vi "Correct_Position_info_7HP.vi"() -> (0 "error out":errorcluster, 4 "Path":path)   [LabVIEW 2018]
panel:
  out "File Changed":bool
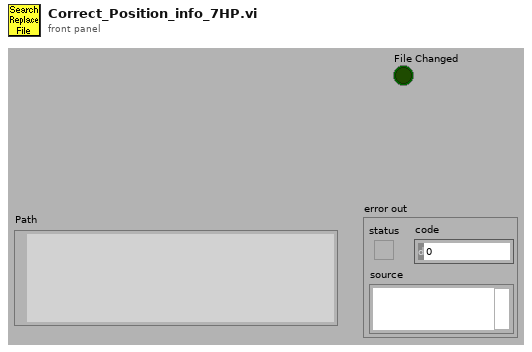
[diagram p1: front panel]
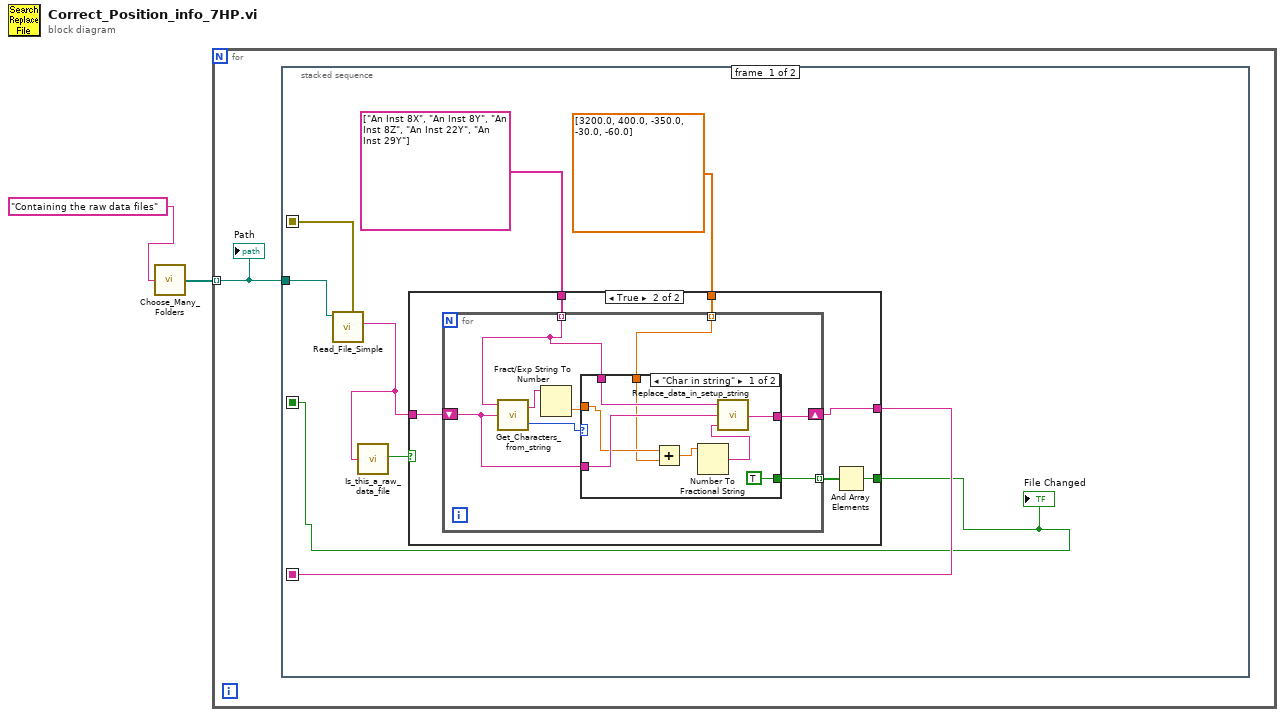
[diagram p0: block diagram]
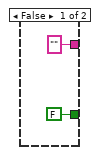
[diagram p2: hidden frame]
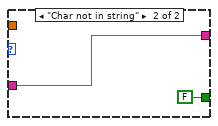
[diagram p3: hidden frame]
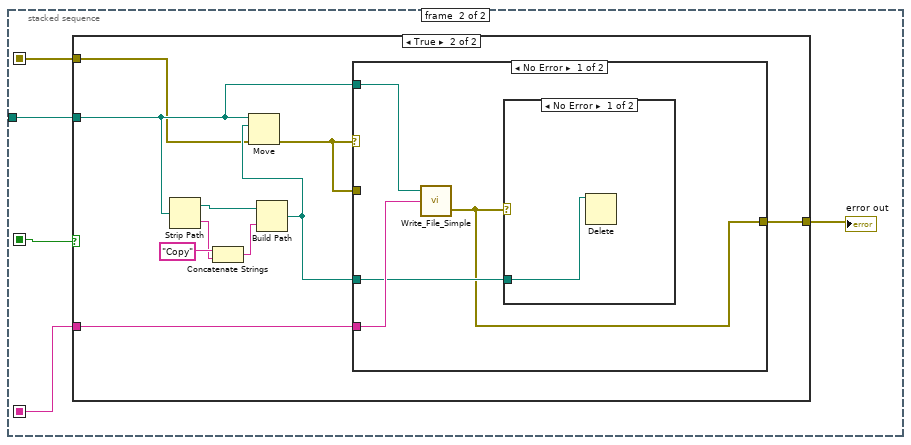
[diagram p4: hidden frame]
diagram:
  n1 = call "Choose_Many_Folders.vi"("Purpose of choosing folder"="Containing the raw data files") -> ("Files"=w1:path[])
  n2 = for {
    tunnel: w1 -> [w3] mode=indexing
    n3 = stacked-sequence {
      seq-local: [w10 _] -> [_ w38]
      seq-local: [w8 _] -> [_ w40]
      seq-local: [w7 _] -> [_ w39]
      tunnel: w3 -> [w11 w42]
      frame #0 {
        n4 = call "Read_File_Simple.vi"("Filename"=w11) -> ("error out"=w10:errorcluster, "string"=w5:string)  [unwired: 4 in, 4 out]
        n5 = call "Is_this_a_raw_data_file.vi"("character string"=w5) -> ("Raw Dat File?"=w6:bool)  [unwired: 2 out]
        n6 = case shown="True" w6 {
          tunnel: string[] ["An Inst 8X", "An Inst 8Y", "An Inst 8Z", "An Inst 22Y", "An Inst 29Y"] -> [_ w19]
          tunnel: ["" ("string") w18] -> w8
          tunnel: w5 -> [_ w17]
          tunnel: [FALSE w15] -> w7
          tunnel: dbl[] [3200.0, 400.0, -350.0, -30.0, -60.0] -> [_ w14]
          frame False {
          }
          frame True {
            n7 = for {
              shift-right: [w26] -> w18
              shift-left: w17 -> [w27]
              tunnel: w19 -> [w21] mode=indexing
              tunnel: [w24] -> w16 mode=indexing
              tunnel: w14 -> [w20] mode=indexing
              n8 = call "Get_Characters_from_string.vi"("Input string"=w27, "Variable name"=w21) -> ("Status"=w25:enum16{"Char in string", "Char not in string"}, "Value"=w23:string)  [unwired: 1 in]
              n9 = Fract/Exp String To Number(string=w23) -> (number=w22:dbl)  [unwired: 3 in, 1 out]
              n10 = case shown="\"Char in string\"" w25 {
                tunnel: w27 -> [w35 w37]
                tunnel: [w29 w37] -> w26
                tunnel: w22 -> [w32 _]
                tunnel: [TRUE FALSE] -> w24
                tunnel: w21 -> [w33 _]
                tunnel: w20 -> [w28 _]
                frame "Char in string" {
                  n11 = Add(x=w32, y=w28) -> (x+y=w31:dbl)
                  n12 = Number To Fractional String(number=w31) -> (F-format string=w30:string)  [unwired: 3 in]
                  n13 = call "Replace_data_in_setup_string.vi"("New data string"=w30, "Input string"=w35, "Variable name"=w33) -> ("Appended string"=w29:string)
                }
                frame "Char not in string" {
                }
              }
            }
            n14 = And Array Elements(Boolean array=w16) -> (logical AND=w15:bool)
          }
        }
        "File Changed" <- w7
      }
      frame #1 {
        n15 = case shown="True" w39 {
          tunnel: w42 -> [_ w49]
          tunnel: w40 -> [_ w48]
          tunnel: [w43 w46] -> w41
          tunnel: w38 -> [w43 w44]
          frame False {
          }
          frame True {
            n16 = Strip Path(path=w49) -> (stripped path=w50:path, name=w52:string)
            n17 = Concatenate Strings("Copy" ("name or relative path"), w52) -> (w51:string)
            n18 = Build Path(base path=w50, name or relative path=w51) -> (appended path=w47:path)
            n19 = Move(source path=w49, error in=w44, 10:w47) -> (error out=w45:errorcluster)  [unwired: 2 in, 2 out]
            n20 = case shown="No Error" w45 {
              tunnel: w49 -> [w57 _]
              tunnel: w48 -> [w56 _]
              tunnel: w47 -> [w55 _]
              tunnel: [w54 w59] -> w46
              tunnel: w45 -> [_ w59]
              frame No Error {
                n21 = call "Write_File_Simple.vi"("character string"=w56, "file path"=w57) -> ("error out"=w54:errorcluster)  [unwired: 1 in, 1 out]
                n22 = case shown="No Error" w54 {
                  tunnel: w55 -> [w58 _]
                  frame No Error {
                    n23 = Delete(path (use dialog)=w58) -> ()  [unwired: 4 in, 3 out]
                  }
                  frame Error {
                  }
                }
              }
              frame Error {
              }
            }
          }
        }
        "error out" <- w41
      }
    }
    "Path" <- w3
  }
